vi "Set GUI Control.vi"(8 "error in (no error)":errorcluster, 10 "GUI Control":refnum<class "GUI Control.lvclass">, 11 "GUI Control Builder in":refnum<class "GUI Control Builder.lvclass">) -> (0 "error out":errorcluster, 3 "GUI Control Builder out":refnum<class "GUI Control Builder.lvclass">)   [LabVIEW 2015, in "GUI Control Builder.lvclass"]
uses:
  GUI Control Builder.lvclass
  GUI Controls/GUI Control/GUI Control.lvclass
  GUI Control Builder.lvclass/GUI Control Builder.ctl
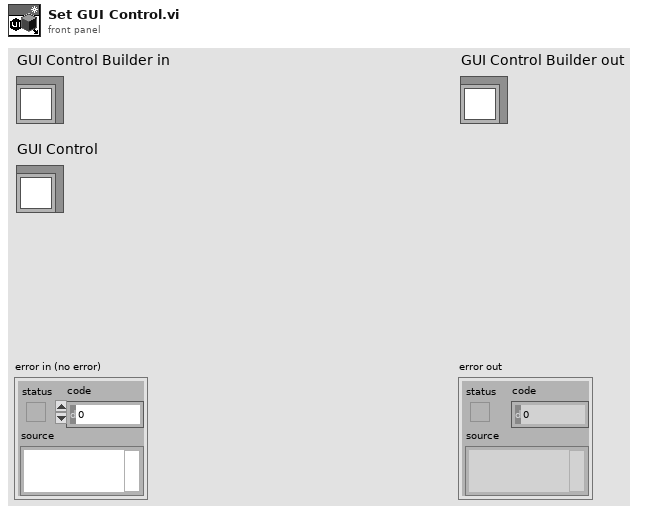
[diagram p1: front panel]
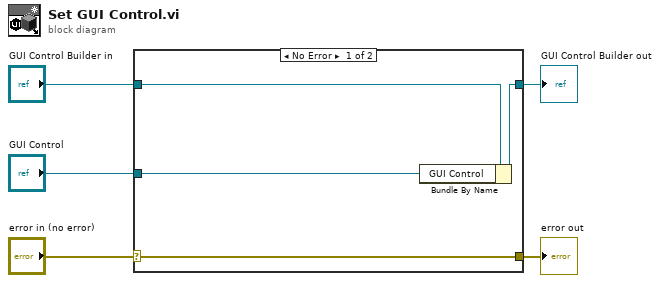
[diagram p0: block diagram]
diagram:
  n1 = case shown="No Error" "error in (no error)" {
    selector: "error in (no error)" -> [w9 w10]
    tunnel: [w9 w10] -> w4
    tunnel: [w7 w11] -> w2
    tunnel: "GUI Control Builder in" -> [w8 w11]
    tunnel: "GUI Control" -> [w6 _]
    frame No Error {
      n2 = Bundle By Name(cluster=w8, "GUI Control"=w6) -> (w7:refnum<class "GUI Control Builder.lvclass">)
    }
    frame Error {
    }
  }
  "error out" <- w4
  "GUI Control Builder out" <- w2
